vi "Data Message_F4.vi"(7 "Parent Index":i32=-1, 8 "error in":errorcluster, 10 "Data":sgl[](array[numeric]), 11 "SECS-II Class in":refnum<class "SECS-II Class.lvclass">) -> (0 "error out":errorcluster, 3 "SECS-II Class out":refnum<class "SECS-II Class.lvclass">)   [LabVIEW 2020, in "SECS Communication.lvlib" / "SECS-II Class.lvclass"]
uses:
  SECS-II Class.lvclass
  SECS-II Class.lvclass/SECS-II Class.ctl
  Message Data.ctl
  Data Item Format.ctl
  Format Code.ctl
  Data To Variant_F4.vi
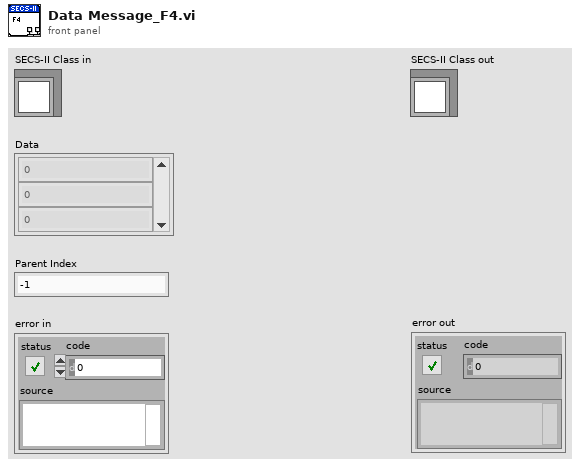
[diagram p1: front panel]
types:
  T1 = typedef "SECS Communication.lvlib/SECS-II Class.lvclass/Data Item Format.ctl" = enum16{"Data Type", "Value"}
  T2 = typedef "SECS Communication.lvlib/SECS-II Class.lvclass/Format Code.ctl" = enum16{"L", "A", "B", "Boolean", "J", "I1", "I2", "I4", "I8", "U1", "U2", "U4", "U8", "F4", "F8", "Char"}
  T3 = typedef "SECS Communication.lvlib/SECS-II Class.lvclass/Message Data.ctl" = cluster{"Index":i32, "Data Item Format":T1, "Format Code":T2, "Parent Index":i32, "Child Index":i32[], "Data":variant}
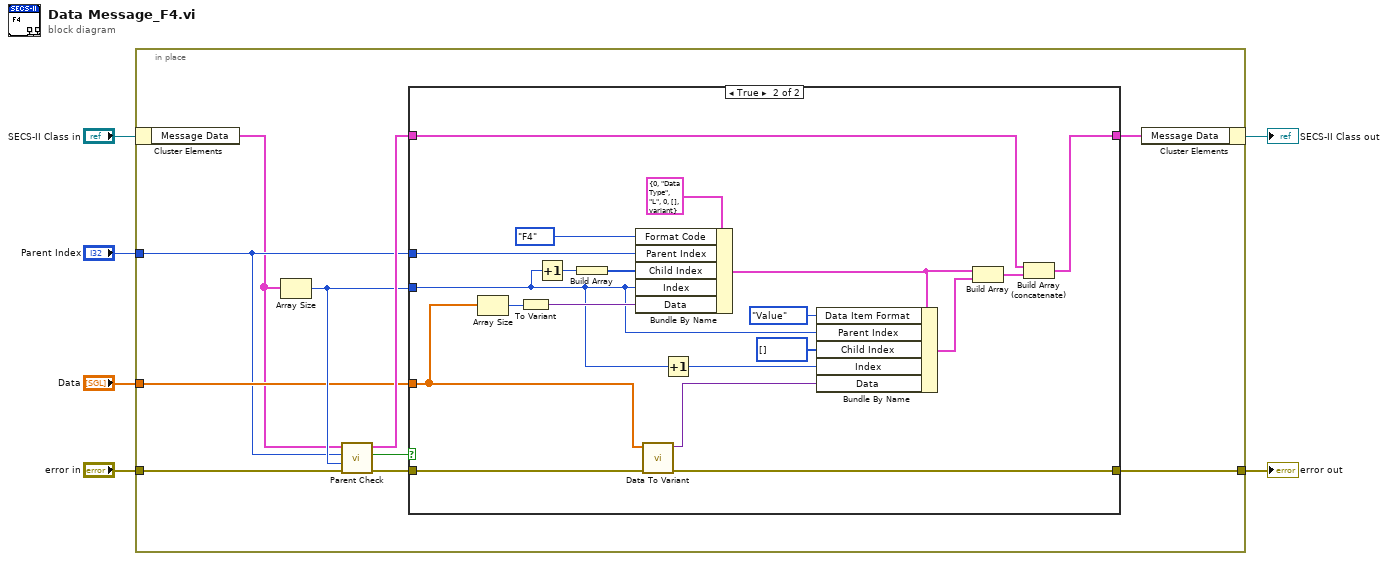
[diagram p0: block diagram]
diagram:
  n1 = in-place {
    in-place-border: "error in" -> [w16]
    in-place-border: [w11] -> w2
    in-place-border: "Data" -> [w10]
    in-place-border: "Parent Index" -> [w9]
    n2 = in-place-cluster #1("SECS-II Class in") -> ("Message Data"=w8:T3[])
    n3 = Array Size(array=w8) -> (size(s)=w12:i32)
    n4 = call "Parent Check.vi"("error in"=w16, "Message Index"=w12, "Parent Index"=w9, "Message Data In"=w8) -> ("error out"=w14:errorcluster, "OK?"=w15:bool, "Message Data Out"=w13:T3[])  [unwired: 5 in]
    n5 = case shown="True" w15 {
      tunnel: w14 -> [w17 w22]
      tunnel: w13 -> [w18 w25]
      tunnel: [w18 w24] -> w7
      tunnel: w9 -> [_ w31]
      tunnel: w12 -> [_ w23]
      tunnel: w10 -> [_ w21]
      tunnel: [w17 w19] -> w11
      frame False {
      }
      frame True {
        n6 = Array Size(array=w21) -> (size(s)=w34:i32)
        n7 = To Variant(anything=w34) -> (Variant=w33:variant)
        n8 = Increment(x=w23) -> (x+1=w36:i32)
        n9 = Build Array(w36) -> (w35:i32[])
        n10 = Bundle By Name(cluster=T3 {"Index"=0, "Data Item Format"=enum."Data Type", "Format Code"=enum."L", "Parent Index"=0, "Child Index"=[], "Data"=variant} ("Message Data"), "Format Code"=Format_Code."F4", "Parent Index"=w31, "Child Index"=w35, "Index"=w23, "Data"=w33) -> (w28:T3)
        n11 = call-poly "Data To Variant.vi"("error in (no error)"=w22, "Data"=w21) -> ("error out"=w19:errorcluster, "Variant"=w20:variant)  [unwired: 8 in]
        n12 = Increment(x=w23) -> (x+1=w29:i32)
        n13 = Bundle By Name(cluster=w28, "Data Item Format"=Data_Item_Format."Value", "Parent Index"=w23, "Child Index"=i32[] [], "Index"=w29, "Data"=w20) -> (w27:T3)
        n14 = Build Array(w28, w27) -> (w26:T3[])
        n15 = Build Array (concatenate)(w25, w26) -> (w24:T3[])
      }
    }
    n16 = in-place-cluster #1("Message Data"=w7) -> (→"SECS-II Class out":refnum<class "SECS-II Class.lvclass">)
  }
  "error out" <- w2
